vi "FTW-Tag-Launch.vi"(5 "FTW Tag Configuration":string="{\n  \"Identity\": \"TagEngine\",\n  \"InboxAddress\": \"inproc://*\",\n  \"LoggerAddress\": \"\",\n  \"Publishers\": {\n    \"TagPublisher\": \"inproc://*\"\n}", 11 "error in":errorcluster) -> (4 "FTW Tag Connector":refnum<class "FTW-ActorConnector.lvclass">, 6 "Tag Address":string, 8 "Publisher Address":string, 15 "error out":errorcluster)   [LabVIEW 2015]
doc: "This method launches a Logger Process which is then referred to based on its LoggerID. Normally in a LabVIEW application, an object's methods would adhere to dataflow with the object wired to the method; however, the Logger Process object likely needs to be accessed by many different portions of your application, and for this reason, it is called by reference, where the LoggerID string refers to the logger.\n\nThis method should be called as one of the very first actions in your application to reasonably ensure the buffer of logged events does not overflow. Events that are logged prior to launching the Logger Process with this method are queued, and will be logged once this process begins."
uses:
  Connector/FTW-ActorConnector.lvclass
  Core/FTW-Tag-Core_Process.vi
  JSON/core/FTW-JSON-Core-EncodingFlags.vi
  JSON/FTW-JSON-Parse.vi
  Reflection/FTW-Reflection-Type.vi
  CodeGen/JSON Deserialize/FTW-JSON-Core-GetFlattenedValue.vi
  CodeGen/JSON Deserialize/FTW-JSON-Deserialize.xnode
  Core/FTW-Tag-Core.lvclass
panel:
  # "Inputs"
  # "Outputs"
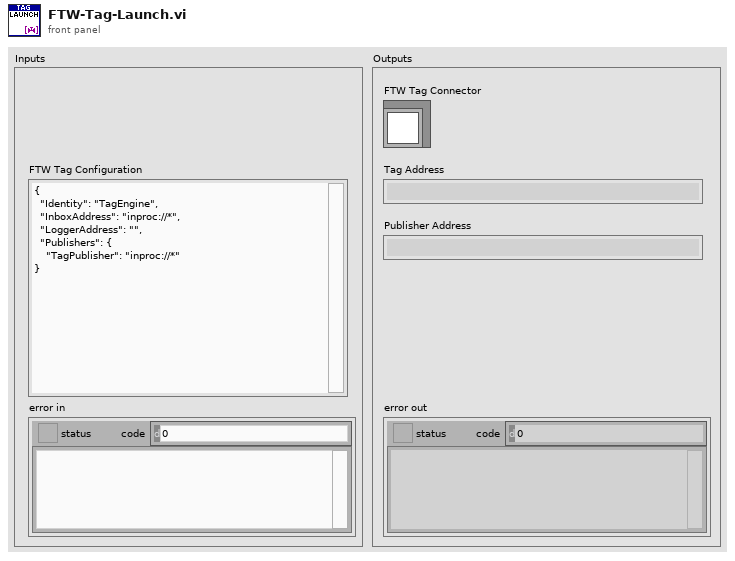
[diagram p1: front panel]
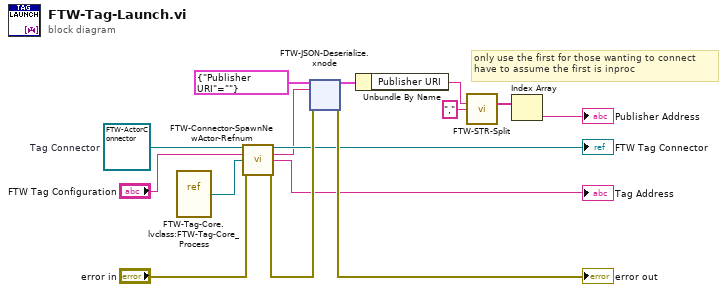
[diagram p0: block diagram]
diagram:
  w11 = refnum<class "FTW-ActorConnector.lvclass"> refnum  # Tag Connector
  # "only use the first for those wanting to connect\nhave to assume the first is inproc"
  n1 = vi-ref "FTW-Tag-Core.lvclass:FTW-Tag-Core_Process.vi"() -> (w8:refnum<vi>)
  n2 = call "FTW-Connector-SpawnNewActor-Refnum.vi"("FTW Actor Connector Type"=w11, "Configuration"="FTW Tag Configuration", "Actor VI Refnum"=w8, "error in"="error in") -> ("FTW Actor Connector"=→"FTW Tag Connector":refnum<class "FTW-ActorConnector.lvclass">, "Initialized Response"=w1:string, "Instance Inbox Address"=→"Tag Address":string, "error out"=w15:errorcluster)  [unwired: 8 in]
  n3 = xnode "FTW-JSON-Deserialize.xnode"("Type and Defaults"=cluster{"Publisher URI":string} {"Publisher URI"=""} ("cluster"), "JSON String"=w1, "error in"=w15) -> ("Values"=w6:cluster{"Publisher URI":string}, "error out"=→"error out":errorcluster)
  n4 = Unbundle By Name(w6) -> ("Publisher URI"=w5:string)
  n5 = call "FTW-STR-Split.vi"("Delimited String"=w5, "Delimiter"=",") -> ("Array of Strings"=w3:string[])  [unwired: 13 in]
  n6 = Index Array(array=w3) -> (element=→"Publisher Address":string)  [unwired: 1 in]
